vi "Get Scalar Charact Result.vi"(11 "error in (no error)":errorcluster) -> (4 "Charact result":T1[](array[typedef]), 15 "error out":errorcluster)   [LabVIEW 2023, in "RFFixtureCharact.Public.lvlib" / "Scalar Path.lvclass"]
uses:
  Scalar Path.lvclass
  Type Definitions/Scalar Charact Result.ctl
  RFFixtureCharact.Public.lvlib
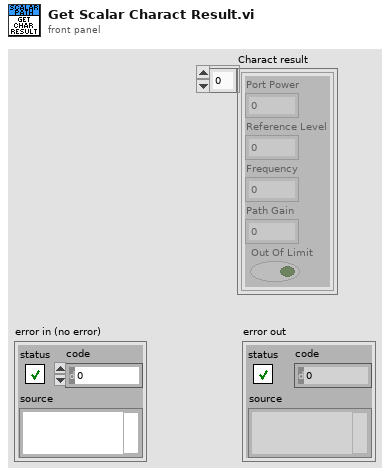
[diagram p1: front panel]
types:
  T1 = typedef "RFFixtureCharact.Public.lvlib/Scalar Path.lvclass/Scalar Charact Result.ctl" = cluster{"Port Power":dbl, "Reference Level":dbl, "Frequency":dbl, "Path Gain":dbl, "Out Of Limit":bool}
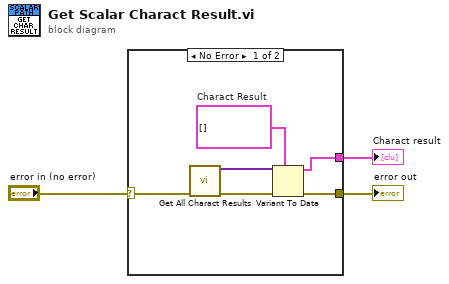
[diagram p0: block diagram]
diagram:
  n1 = case shown="No Error" "error in (no error)" {
    selector: "error in (no error)" -> [w5 w10]
    tunnel: [w8 w10] -> w2
    tunnel: [w7 _] -> w1
    frame No Error {
      w9 = T1[] []  # Charact Result
      n2 = call "Get All Charact Results.vi"("error in"=w5) -> ("All Cal Results"=w6:variant[], "error out"=w4:errorcluster)  [unwired: 13 in]
      n3 = Variant To Data(error in=w4, type=w9, Variant=w6) -> (data=w7:T1[], error out=w8:errorcluster)
    }
    frame Error {
    }
  }
  "error out" <- w2
  "Charact result" <- w1
